vi "PORT.vi"(3 "error INPUT":errorcluster, 4 "PIOs output":i8=1 min=0 max=3 step=1 format="%x", 5 "VISA resource Input":refnum<visa-resource-name>) -> (0 "error out":errorcluster, 1 "Value":u8, 2 "VISA resource name out":refnum<visa-resource-name>)   [LabVIEW 2011]
panel:
  out "unsigned byte array":u8[](array[numeric])
  out "x+y":dbl
  out "Read PORT command":u8[](array[numeric])
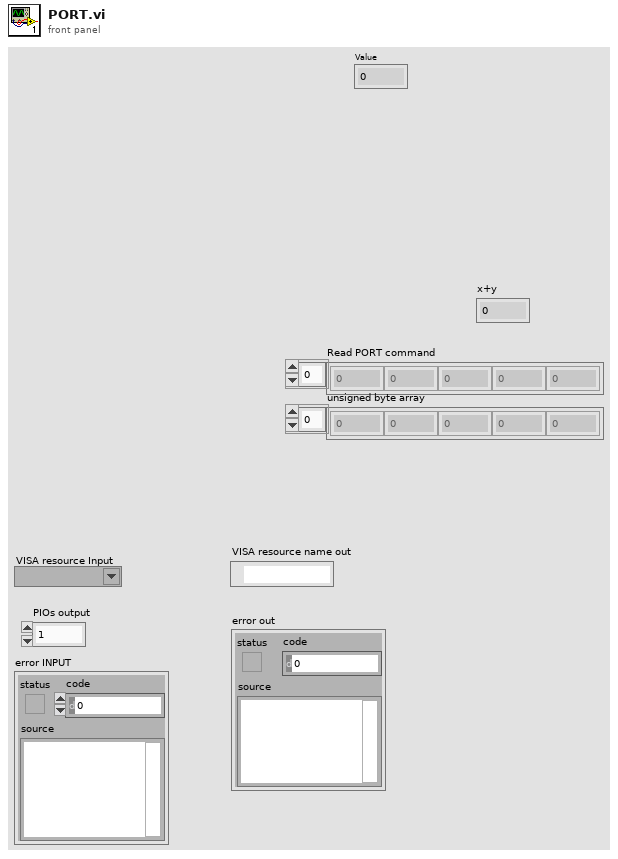
[diagram p1: front panel]
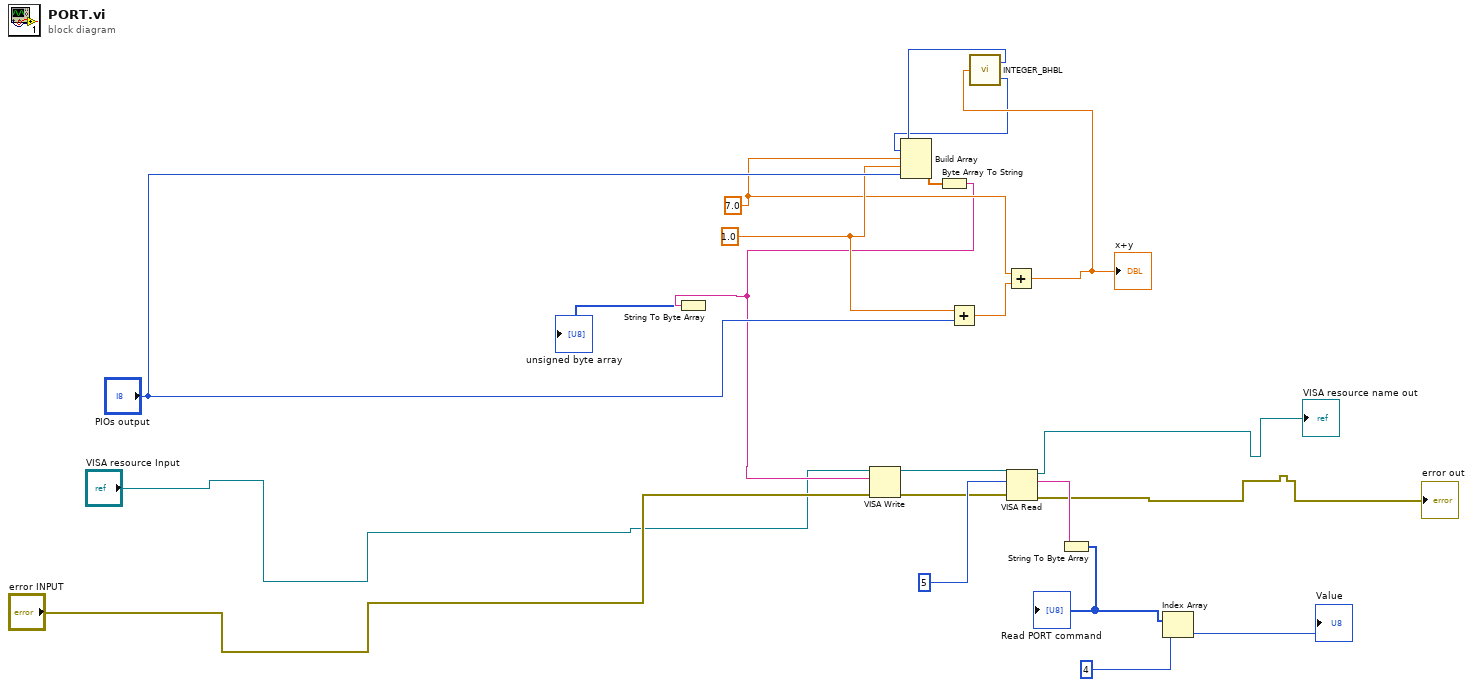
[diagram p0: block diagram]
diagram:
  w14 = 1.0 ("element")
  w12 = 7.0 ("element")
  n1 = Add(x=w14, y="PIOs output") -> (x+y=w13:dbl)
  n2 = Add(x=w12, y=w13) -> (x+y=w11:dbl)
  "x+y" <- w11
  n3 = call "INTEGER_BHBL.vi"("int16"=w11) -> ("Lvalue"=w9:u8, "HValue"=w10:u8)
  n4 = Build Array(w10, w9, w12, w14, "PIOs output") -> (w16:dbl[])
  n5 = Byte Array To String(unsigned byte array=w16) -> (string=w8:string)
  n6 = String To Byte Array(string=w8) -> (unsigned byte array=→"unsigned byte array":u8[])
  n7 = VISA Write(VISA resource name="VISA resource Input", write buffer=w8, error in (no error)="error INPUT") -> (VISA resource name out=w17:refnum<visa-resource-name>, error out=w18:errorcluster)  [unwired: 1 out]
  n8 = VISA Read(VISA resource name=w17, byte count=u32 5, error in (no error)=w18) -> (VISA resource name out=→"VISA resource name out":refnum<visa-resource-name>, read buffer=w19:string, error out=→"error out":errorcluster)  [unwired: 1 out]
  n9 = String To Byte Array(string=w19) -> (unsigned byte array=w3:u8[])
  "Read PORT command" <- w3
  n10 = Index Array(array=w3, index=4) -> (element=→"Value":u8)
